vi "SMTP Email [RCPT].vi"(4 "error in (no error)":errorcluster, 6 "address":string, 7 "smtp session":T1) -> (0 "error out":errorcluster, 1 "reply":string, 2 "reply code":i32, 3 "smtp session out":T1)   [LabVIEW 2011, in "NewNI_SMTPEmail.lvlib"]
doc: "Sends the RCPT command to the SMTP server through TCP connection described by \"connection ID\", receives reply and interprets it.\n\nReciever's e-mail: E-mail address of the person (or mailbox) you want to send your mail.\n\nThis VI returns \"connection ID out,\" and the results of the error interpretation to the \"error out\" cluster."
uses:
  NewNI_SMTPEmail.lvlib
  SMTP Email Session.ctl
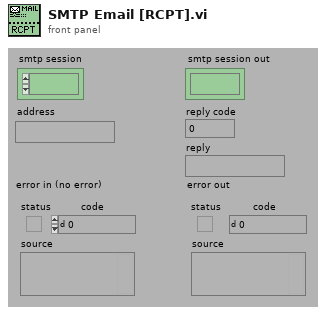
[diagram p1: front panel]
types:
  T1 = typedef "NewNI_SMTPEmail.lvlib/SMTP Email Session.ctl" = refnum<k1>
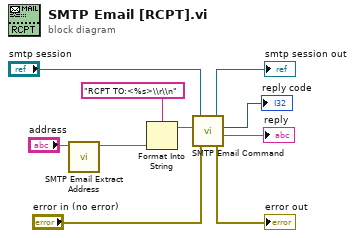
[diagram p0: block diagram]
diagram:
  n1 = call "SMTP Email Extract Address.vi"("string with address"="address") -> ("address"=w1:string)  [unwired: 6 out]
  n2 = Format Into String(format string="RCPT TO:<%s>\\r\\n", w1) -> (resulting string=w3:string)  [unwired: 2 in, 1 out]
  n3 = call "SMTP Email Command.vi"("error in (no error)"="error in (no error)", "command"=w3, "smtp session"="smtp session") -> ("error out"=→"error out":errorcluster, "reply"=→"reply":string, "reply code"=→"reply code":i32, "smtp session out"=→"smtp session out":T1)  [unwired: 1 in]
